vi "ke2000 Action Abort Trigger.vi"(0 "VISA resource name":refnum<visa-resource-name>, 5 "error in (no error)":errorcluster) -> (14 "VISA resource name out":refnum<visa-resource-name>, 19 "error out":errorcluster)   [LabVIEW 2010]
doc: "This VI aborts the trigger sequence of the instrument and causes it to go into an idle state."
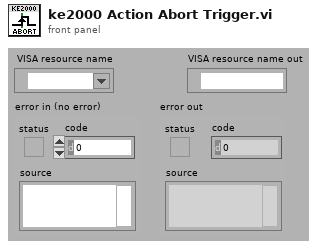
[diagram p1: front panel]
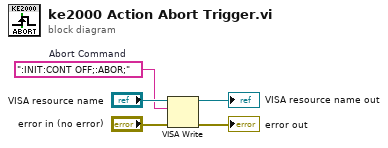
[diagram p0: block diagram]
diagram:
  w1 = ":INIT:CONT OFF;:ABOR;"  # Abort Command
  n1 = VISA Write(VISA resource name="VISA resource name", write buffer=w1, error in (no error)="error in (no error)") -> (VISA resource name out=→"VISA resource name out":refnum<visa-resource-name>, error out=→"error out":errorcluster)  [unwired: 1 out]
